vi "Write Nipkg Metadata.vi"(7 "64-bit?":bool, 8 "Error In":errorcluster, 9 "Package Version":string="0.2.0", 10 "LabVIEW Version":u16=2014, 11 "Root Folder":path) -> (0 "Error Out":errorcluster)   [LabVIEW 2014]
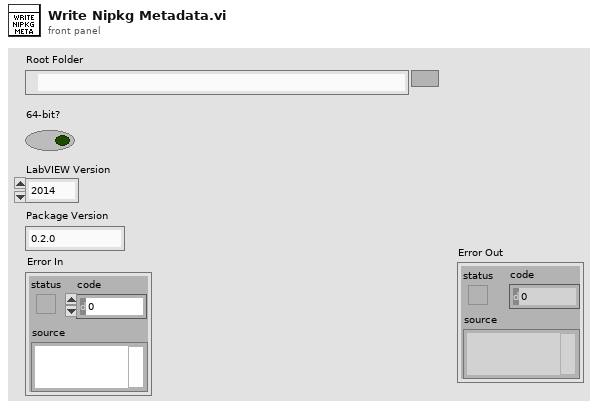
[diagram p1: front panel]
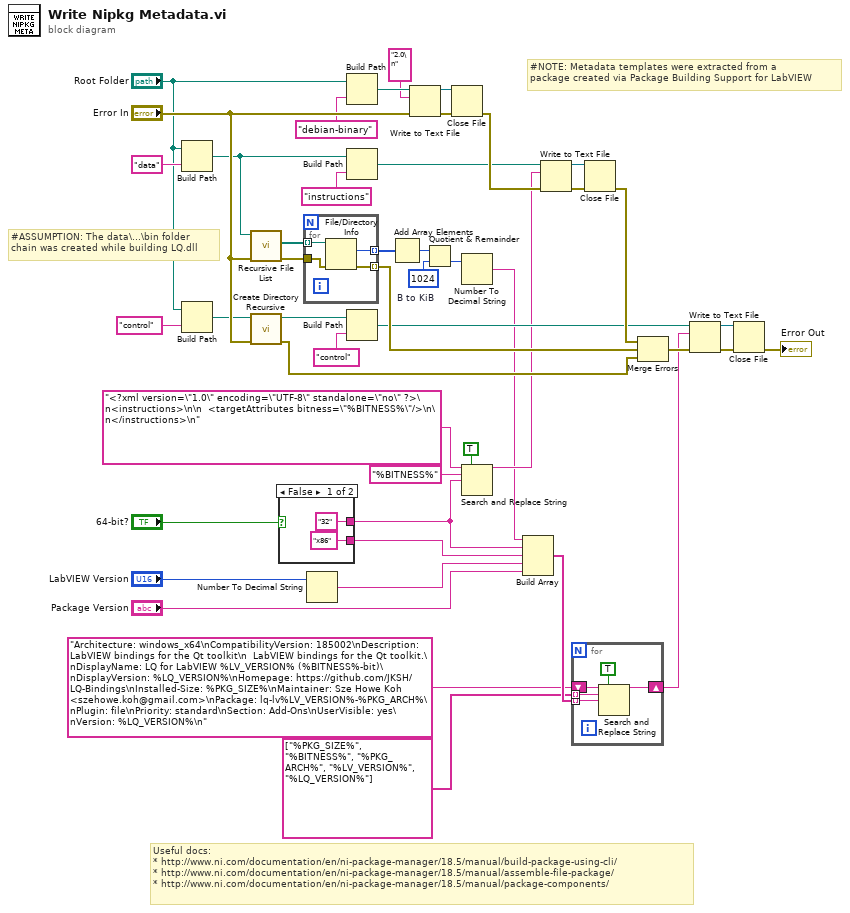
[diagram p0: block diagram]
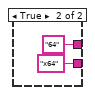
[diagram p2: hidden frame]
diagram:
  w9 = i64 1024  # B to KiB
  # "Useful docs:\n* http://www.ni.com/documentation/en/ni-package-manager/18.5/manual/build-package-using-cli/\n* http://www.ni.com/documentation/en/ni-package-manager/18.5/manual/assemble-file-package/\n* http://www.ni.com/documentation/en/ni-package-manager/18.5/manual/package-components/"
  # "#ASSUMPTION: The data\\...\\bin folder\nchain was created while building LQ.dll"
  # "#NOTE: Metadata templates were extracted from a\npackage created via Package Building Support for LabVIEW"
  n1 = Build Path(base path="Root Folder", name or relative path="data") -> (appended path=w7:path)
  n2 = Build Path(base path="Root Folder", name or relative path="control") -> (appended path=w38:path)
  n3 = call <vilib>:"Recursive File List.vi"("error in (no error)"="Error In", "Folder Path"=w7) -> ("error out"=w6:errorcluster, "All Files in Dir"=w12:path[])  [unwired: 5 in, 3 out]
  n4 = call <vilib>:"Create Directory Recursive.vi"("error in (no error)"="Error In", "directory"=w38) -> ("error out"=w47:errorcluster, "directory copy"=w36:path)  [unwired: 3 in, 1 out]
  n5 = case shown="False" "64-bit?" {
    tunnel: ["32" "64"] -> w22
    tunnel: ["x86" "x64"] -> w21
    frame False {
    }
    frame True {
    }
  }
  n6 = for {
    tunnel: w12 -> [w55] mode=indexing
    tunnel: [w54] -> w11 mode=indexing
    tunnel: w6 -> [w53]
    tunnel: [w52] -> w45 mode=indexing
    n7 = File/Directory Info(path=w55, error in=w53) -> (size=w54:i64, error out=w52:errorcluster)  [unwired: 5 out]
  }
  n8 = Number To Decimal String(number="LabVIEW Version") -> (decimal integer string=w20:string)  [unwired: 1 in]
  n9 = Build Path(base path="Root Folder", name or relative path="debian-binary") -> (appended path=w32:path)
  n10 = Build Path(base path=w7, name or relative path="instructions") -> (appended path=w30:path)
  n11 = Build Path(base path=w36, name or relative path="control") -> (appended path=w31:path)
  n12 = Add Array Elements(numeric array=w11) -> (sum=w10:i64)
  n13 = Write to Text File(file (use dialog)=w32, text="2.0\n", error in="Error In") -> (refnum out=w18:refnum<file>, error out=w17:errorcluster)  [unwired: 1 in, 1 out]
  n14 = Quotient & Remainder(x=w10, y=w9) -> (floor(x/y)=w8:i64)  [unwired: 1 out]
  n15 = Close File(refnum=w18, error in=w17) -> (error out=w42:errorcluster)  [unwired: 1 out]
  n16 = Number To Decimal String(number=w8) -> (decimal integer string=w1:string)  [unwired: 1 in]
  n17 = Search and Replace String(replace all?=TRUE ("replace all? (F)"), input string="<?xml version=\"1.0\" encoding=\"UTF-8\" standalone=\"no\" ?>\n<instructions>\n\n  <targetAttributes bitness=\"%BITNESS%\"/>\n\n</instructions>\n", search string="%BITNESS%", replace string=w22) -> (result string=w3:string)  [unwired: 4 in, 3 out]
  n18 = Build Array(w1, w22, w21, w20, "Package Version") -> (w41:string[])
  n19 = Write to Text File(file (use dialog)=w30, text=w3, error in=w42) -> (refnum out=w14:refnum<file>, error out=w13:errorcluster)  [unwired: 1 in, 1 out]
  n20 = for {
    tunnel: w41 -> [w58] mode=indexing
    tunnel: string[] ["%PKG_SIZE%", "%BITNESS%", "%PKG_ARCH%", "%LV_VERSION%", "%LQ_VERSION%"] -> [w57] mode=indexing
    shift-right: [w56] -> w4
    shift-left: "Architecture: windows_x64\nCompatibilityVersion: 185002\nDescription: LabVIEW bindings for the Qt toolkit\n  LabVIEW bindings for the Qt toolkit.\nDisplayName: LQ for LabVIEW %LV_VERSION% (%BITNESS%-bit)\nDisplayVersion: %LQ_VERSION%\nHomepage: https://github.com/JKSH/LQ-Bindings\nInstalled-Size: %PKG_SIZE%\nMaintainer: Sze Howe Koh <szehowe.koh@gmail.com>\nPackage: lq-lv%LV_VERSION%-%PKG_ARCH%\nPlugin: file\nPriority: standard\nSection: Add-Ons\nUserVisible: yes\nVersion: %LQ_VERSION%\n" -> [w59]
    n21 = Search and Replace String(replace all?=TRUE ("replace all? (F)"), input string=w59, search string=w57, replace string=w58) -> (result string=w56:string)  [unwired: 4 in, 3 out]
  }
  n22 = Close File(refnum=w14, error in=w13) -> (error out=w46:errorcluster)  [unwired: 1 out]
  n23 = Merge Errors(w46, w45, w47) -> (w43:errorcluster)
  n24 = Write to Text File(file (use dialog)=w31, text=w4, error in=w43) -> (refnum out=w16:refnum<file>, error out=w15:errorcluster)  [unwired: 1 in, 1 out]
  n25 = Close File(refnum=w16, error in=w15) -> (error out=→"Error Out":errorcluster)  [unwired: 1 out]
